vi "APS set feeder point 2D.vi"(7 "LastFlag":i32, 8 "error in (no error)":errorcluster caption="错误输入（无错误）", 9 "Size":i32, 10 "PtArray":T1, 11 "GroupId":i32) -> (0 "error out":errorcluster caption="错误输出", 2 "PtArray out":T1, 3 "function return":i32)   [LabVIEW 2011, in "APS168.lvlib"]
doc: "I32 FNTYPE APS_set_feeder_point_2D( I32 GroupId, PNT_DATA_2D* PtArray, I32 Size, I32 LastFlag );"
uses:
  APS168.lvlib
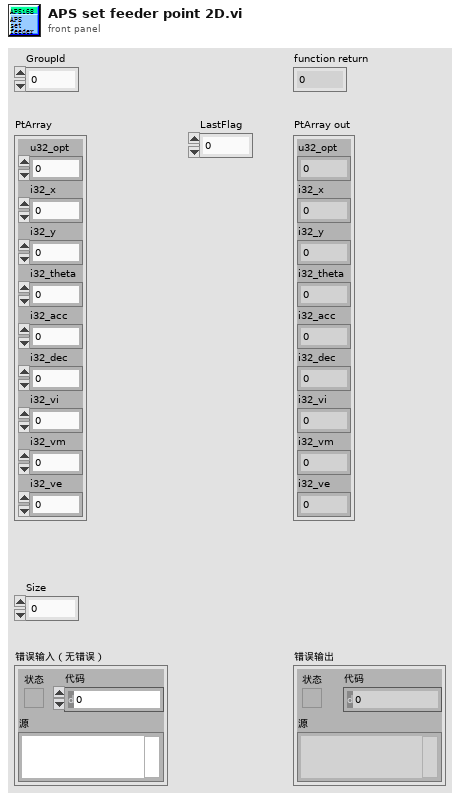
[diagram p1: front panel]
types:
  T1 = cluster{"u32_opt":u32, "i32_x":i32, "i32_y":i32, "i32_theta":i32, "i32_acc":i32, "i32_dec":i32, "i32_vi":i32, "i32_vm":i32, "i32_ve":i32}
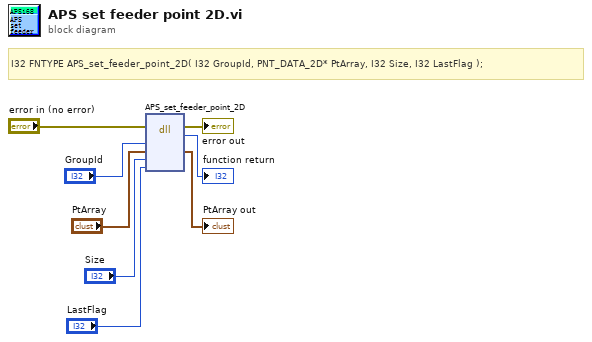
[diagram p0: block diagram]
diagram:
  # "I32 FNTYPE APS_set_feeder_point_2D( I32 GroupId, PNT_DATA_2D* PtArray, I32 Size, I32 LastFlag );"
  n1 = dll-call lib="PTH1Labs E软件ADLINK 204CAPS_1_7_1_LIB line 连续运动204APS168.*" fn="APS_set_feeder_point_2D"(error in="error in (no error)", "GroupId"="GroupId", "PtArray"="PtArray", "Size"="Size", "LastFlag"="LastFlag") -> (error out=→"error out":errorcluster, →"function return":i32, "PtArray"=→"PtArray out":T1)  [unwired: 5 in, 1 out]
